vi "DoDrawTiles.vi"(8 "error in (no error)":errorcluster, 10 "TilesLoopData in":T2, 11 "Refnum in":T1) -> (0 "error out":errorcluster, 3 "TilesLoopData out":T2)   [LabVIEW 2019, in "RT_Game.lvlib" / "Engine.lvclass"]
uses:
  Engine.lvclass
  TilesLoopData.ctl
  Coordinate.ctl
  SlideJob.ctl
  ScreenSide.ctl
  FPGA_Interface.ctl
  <vilib>/Utility/error.llb/Error Cluster From Error Code.vi
  <vilib>/rvi/errors/niLvFpgaAdjustHostInterfaceError.vi
  <vilib>/rvi/interface/nirviMethod/nirviMethod.xnode
  FPGA Bitfiles/myriogameconsole_FPGATarget_Main_ntsPRcBZGxk.lvbitx
  <vilib>/FPGAPlugInAG/myRIO-1900/niLvFpga_WriteFifo_myRIO-1900.vi
  <vilib>/rvi/errors/niLvFpgaMergeErrorWithErrorCode.vi
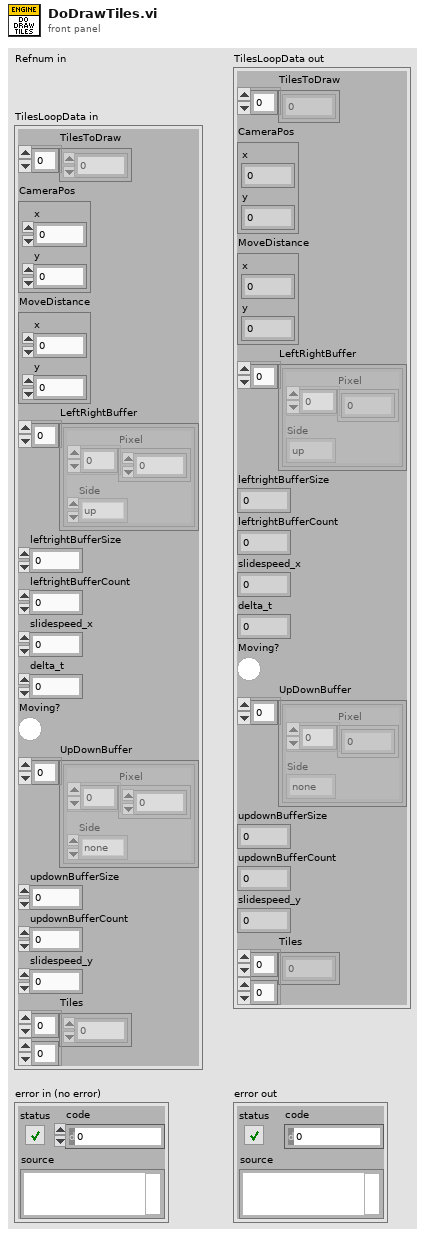
[diagram p1: front panel]
types:
  T1 = typedef "FPGA_Interface.ctl" = refnum<k20>
  T2 = typedef "RT_Game.lvlib/Engine.lvclass/TilesLoopData.ctl" = cluster{"TilesToDraw":u64[], "CameraPos":T3, "MoveDistance":T3, "LeftRightBuffer":T4[], "leftrightBufferSize":i16, "leftrightBufferCount":i16, "slidespeed_x":dbl, "delta_t":dbl, "Moving?":bool, "UpDownBuffer":T4[], "updownBufferSize":i16, "updownBufferCount":i16, "slidespeed_y":dbl, "Tiles":u32[][]}
  T3 = typedef "RT_Game.lvlib/Engine.lvclass/Coordinate.ctl" = cluster{"x":dbl, "y":dbl}
  T4 = typedef "RT_Game.lvlib/Engine.lvclass/SlideJob.ctl" = cluster{"Pixel":u32[], "Side":T5}
  T5 = typedef "RT_Game.lvlib/Engine.lvclass/ScreenSide.ctl" = enum16{"up", "down", "left", "right", "none"}
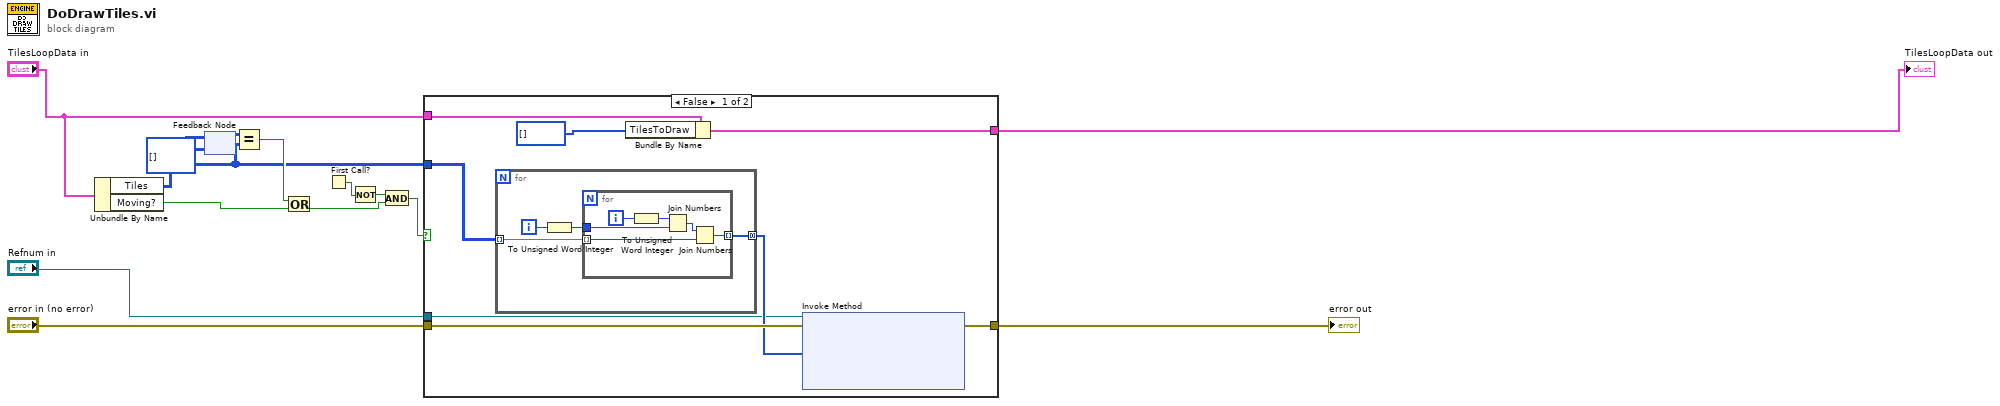
[diagram p0: block diagram]
diagram:
  n1 = Unbundle By Name("TilesLoopData in") -> ("Tiles"=w1:u32[][], "Moving?"=w12:bool)
  n2 = feedback-in #1(w1) -> ()
  n3 = feedback #1(u32[][] [] ("Tiles")) -> (w2:u32[][])
  n4 = Equal?(x=w2, y=w1) -> (x = y?=w3:bool)
  n5 = Or(x=w3, y=w12) -> (x .or. y?=w4:bool)
  n6 = First Call?() -> (First Call?: T/F=w13:bool)
  n7 = Not(x=w13) -> (.not. x?=w14:bool)
  n8 = And(x=w14, y=w4) -> (x .and. y?=w6:bool)
  n9 = case shown="False" w6 {
    tunnel: "error in (no error)" -> [w22 w34]
    tunnel: "Refnum in" -> [w20 _]
    tunnel: [w19 w34] -> w11
    tunnel: w1 -> [w18 _]
    tunnel: "TilesLoopData in" -> [w17 w33]
    tunnel: [w16 w33] -> w7
    frame False {
      n10 = for {
        tunnel: w18 -> [w26] mode=indexing
        tunnel: [w23] -> w21 mode=concatenating
        i -> [w25]
        n11 = To Unsigned Word Integer(number=w25) -> (unsigned 16bit integer=w24:u16)
        n12 = for {
          tunnel: w26 -> [w29] mode=indexing
          tunnel: w24 -> [w30]
          tunnel: [w27] -> w23 mode=indexing
          i -> [w32]
          n13 = To Unsigned Word Integer(number=w32) -> (unsigned 16bit integer=w31:u16)
          n14 = Join Numbers(hi=w31, lo=w30) -> ((hi.lo)=w28:u32)
          n15 = Join Numbers(hi=w28, lo=w29) -> ((hi.lo)=w27:u64)
        }
      }
      n16 = Bundle By Name(cluster=w17, "TilesToDraw"=u64[] []) -> (w16:T2)
      n17 = xnode "Invoke Method"("FPGA VI Reference In"=w20, "error in"=w22, "Data"=w21) -> ("error out"=w19:errorcluster)  [unwired: 1 in, 2 out]
    }
    frame True {
    }
  }
  "TilesLoopData out" <- w7
  "error out" <- w11
